vi "Init.vi"(7 "Sender":refnum<class "Sender.lvclass">, 9 "Error":errorcluster, 10 "Actor":refnum<class "Actor.lvclass">) -> (3 "Terminated Msg out":refnum<class "Terminated Msg.lvclass">)   [LabVIEW 2025, in "jettl.lvlib" / "Terminated Msg.lvlib" / "Terminated Msg.lvclass"]
uses:
  Terminated Msg.lvclass
  Terminated Msg.lvclass/Terminated Msg.ctl
  Actor/Actor/Actor.lvclass
  Sender/Sender/Sender.lvclass
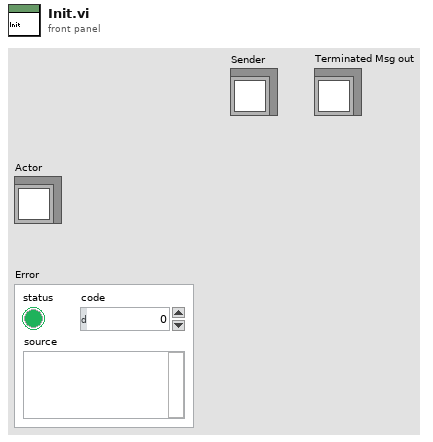
[diagram p1: front panel]
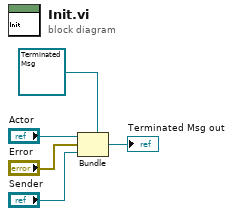
[diagram p0: block diagram]
diagram:
  n1 = Bundle "Bundle"(cluster=refnum<class "Terminated Msg.lvclass"> refnum ("Last Ack Creator Queue Msg Strategy out"), "Actor", "Error", "Sender") -> (→"Terminated Msg out":refnum<class "Terminated Msg.lvclass">)
